vi "Main.vi"   [LabVIEW 2018]
uses:
  Journal/Journal.lvclass
  Persistence/Persistence.lvclass
  Journal/Journal.lvclass/Journal.ctl
  <vilib>/Utility/error.llb/Clear Errors.vi
  <vilib>/Platform/browser.llb/Open URL in Default Browser (path).vi
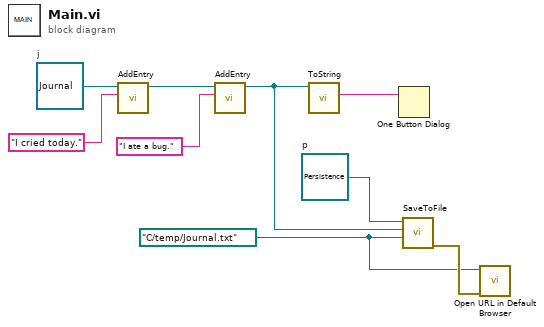
[diagram p0: block diagram]
diagram:
  w2 = refnum<class "Persistence.lvclass"> refnum  # p
  w1 = path "C:/temp/Journal.txt" ("File Path")
  w9 = refnum<class "Journal.lvclass"> refnum  # j
  n1 = call "AddEntry.vi"("Entry"="I cried today.", "Journal In"=w9) -> ("Journal Out"=w7:refnum<class "Journal.lvclass">)  [unwired: 8 in, 1 out]
  n2 = call "AddEntry.vi"("Entry"="I ate a bug.", "Journal In"=w7) -> ("Journal Out"=w3:refnum<class "Journal.lvclass">)  [unwired: 8 in, 1 out]
  n3 = call "ToString.vi"("Journal In"=w3) -> ("String"=w5:string)  [unwired: 9 in, 1 out]
  n4 = One Button Dialog(message=w5) -> ()  [unwired: 1 in, 1 out]
  n5 = call "SaveToFile.vi"("File Path"=w1, "Journal"=w3, "Persistance"=w2) -> ("Error Out"=w4:errorcluster)  [unwired: 8 in]
  n6 = call-poly <vilib>:"Open URL in Default Browser.vi"("error in (no error)"=w4, "path"=w1) -> ()  [unwired: 4 in, 2 out]
